vi "Load and Save Config Example.vi"() -> ()   [LabVIEW 2021]
uses:
  RWC_Actions.ctl
panel:
  in  "Cancel":bool
  in  "OK":bool
  in  "Numeric Option 2":dbl
  in  "Numeric Option 1":dbl
  in  "Option 4":bool
  in  "Option 3":bool
  in  "Option 2":bool
  in  "Option 1":bool
  in  "User":u16(ring) items=["John", "Paul", "George", "Ringo"]
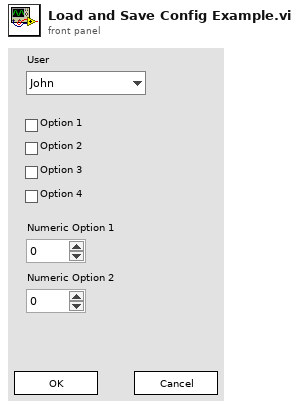
[diagram p1: front panel]
types:
  T1 = typedef "RWC_Actions.ctl" = enum16{"Read", "Write", "Read and Create"}
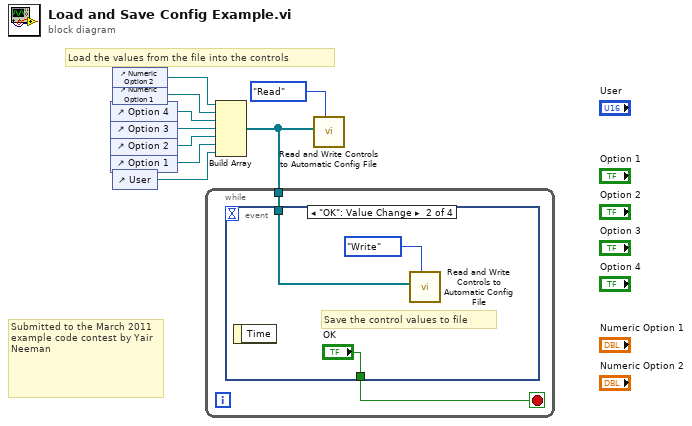
[diagram p0: block diagram]
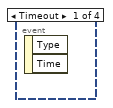
[diagram p2: hidden frame]
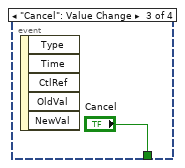
[diagram p3: hidden frame]
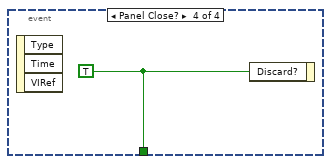
[diagram p4: hidden frame]
diagram:
  # "Submitted to the March 2011 example code contest by Yair Neeman"
  # "Load the values from the file into the controls"
  n1 = control-ref of="Option 4"() -> (w7:refnum<vi>)
  n2 = control-ref of="Option 3"() -> (w6:refnum<vi>)
  n3 = control-ref of="Option 2"() -> (w5:refnum<vi>)
  n4 = control-ref of="Option 1"() -> (w4:refnum<vi>)
  n5 = control-ref of="Numeric Option 2"() -> (w9:refnum<vi>)
  n6 = control-ref of="Numeric Option 1"() -> (w8:refnum<vi>)
  n7 = control-ref of="User"() -> (w3:refnum<vi>)
  n8 = Build Array(w9, w8, w7, w6, w5, w4, w3) -> (w1:refnum<vi>[])
  n9 = while {
    tunnel: w1 -> [w10]
    stop <- w11 stop-if-true
    n10 = event shown="[1] \"OK\": Value Change" {
      selector: _ -> [_ _ _ _]
      dyn-events: _ -> [_ _ _ _]
      timeout: _ -> [_ _ _ _]
      tunnel: [_ "OK" "Cancel" w16] -> w11
      tunnel: w10 -> [_ w12 _ _]
      event Timeout {
        n11 = event-data() -> ()  [unwired: 1 in, 2 out]
      }
      event "OK": Value Change {
        # "Save the control values to file"
        n12 = event-data() -> ()  [unwired: 1 in, 1 out]
        n13 = call "Read and Write Controls to Automatic Config File.vi"("Action"=RWC_Actions."Write", "Control References"=w12) -> ()  [unwired: 9 in, 1 out]
      }
      event "Cancel": Value Change {
        n14 = event-data() -> ()  [unwired: 1 in, 5 out]
      }
      event Panel Close? {
        w16 = TRUE
        n15 = event-data() -> ()  [unwired: 1 in, 3 out]
        n16 = event-data("Discard?"=w16) -> ()  [unwired: 1 in, 1 out]
      }
    }
  }
  n17 = call "Read and Write Controls to Automatic Config File.vi"("Action"=RWC_Actions."Read", "Control References"=w1) -> ()  [unwired: 9 in, 1 out]
